vi "New TDMS Channel Group.vi"(8 "error in (no error)":errorcluster, 11 "TDMS Channel Group":T2={"Group Name"="", "Group Description"="", "Group Properties"=[], "Channels"=[], "Time Channel Options"=enum."No Time Channel", "Time Channel Name"="Time"}) -> (0 "error out":errorcluster, 3 "TdmsChannelGroup Ref":T1)   [LabVIEW 2020, in "NI_VS Data Logging API.lvlib"]
doc: "Creates a TdmsChannelGroup object based on the settings of the <b>TDMS Channel Group</b> input."
uses:
  <vilib>/NI VeriStand/Execution/DataLogging/NI_VS Data Logging API.lvlib
  <vilib>/NI VeriStand/Execution/DataLogging/TDMS Channel Group.ctl
  <vilib>/NI VeriStand/Execution/DataLogging/TDMS Property.ctl
  <vilib>/NI VeriStand/Execution/DataLogging/TDMS Channel.ctl
  <vilib>/NI VeriStand/Execution/DataLogging/Time Channel Options.ctl
  <vilib>/NI VeriStand/Execution/DataLogging/TdmsChannelGroup Ref.ctl
  NationalInstruments.VeriStand.ClientAPI
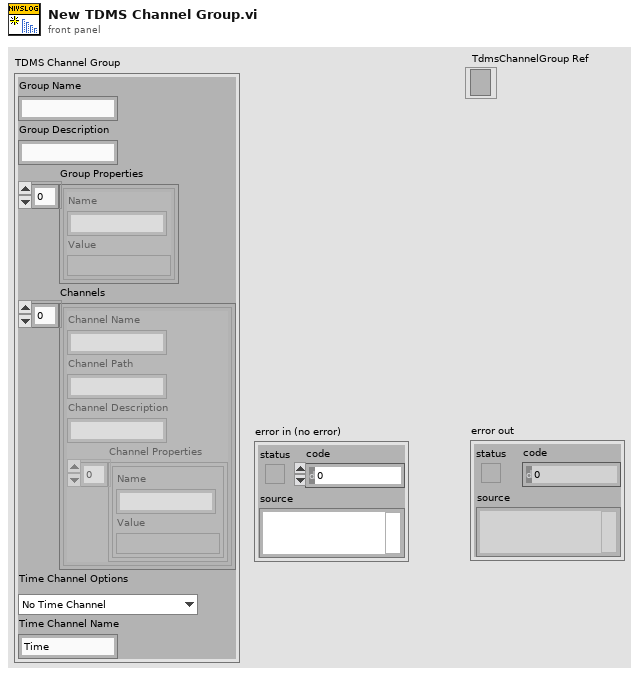
[diagram p1: front panel]
types:
  T1 = typedef "NI_VS Data Logging API.lvlib/TdmsChannelGroup Ref.ctl" = refnum<k24>
  T2 = typedef "NI_VS Data Logging API.lvlib/TDMS Channel Group.ctl" = cluster{"Group Name":string, "Group Description":string, "Group Properties":T3[], "Channels":T4[], "Time Channel Options":T5, "Time Channel Name":string}
  T3 = typedef "NI_VS Data Logging API.lvlib/TDMS Property.ctl" = cluster{"Name":string, "Value":variant}
  T4 = typedef "NI_VS Data Logging API.lvlib/TDMS Channel.ctl" = cluster{"Channel Name":string, "Channel Path":string, "Channel Description":string, "Channel Properties":T3[]}
  T5 = typedef "NI_VS Data Logging API.lvlib/Time Channel Options.ctl" = enum16{"No Time Channel", "Absolute Time", "System Time", "System Time - Microseconds", "Absolute Time as Double", "Relative To First Start Trigger", "Relative To Session Start"}
  T6 = typedef "NI_VS Data Logging API.lvlib/TdmsProperty Ref.ctl" = refnum<k24>
  T7 = typedef "NI_VS Data Logging API.lvlib/TdmsChannel Ref.ctl" = refnum<k24>
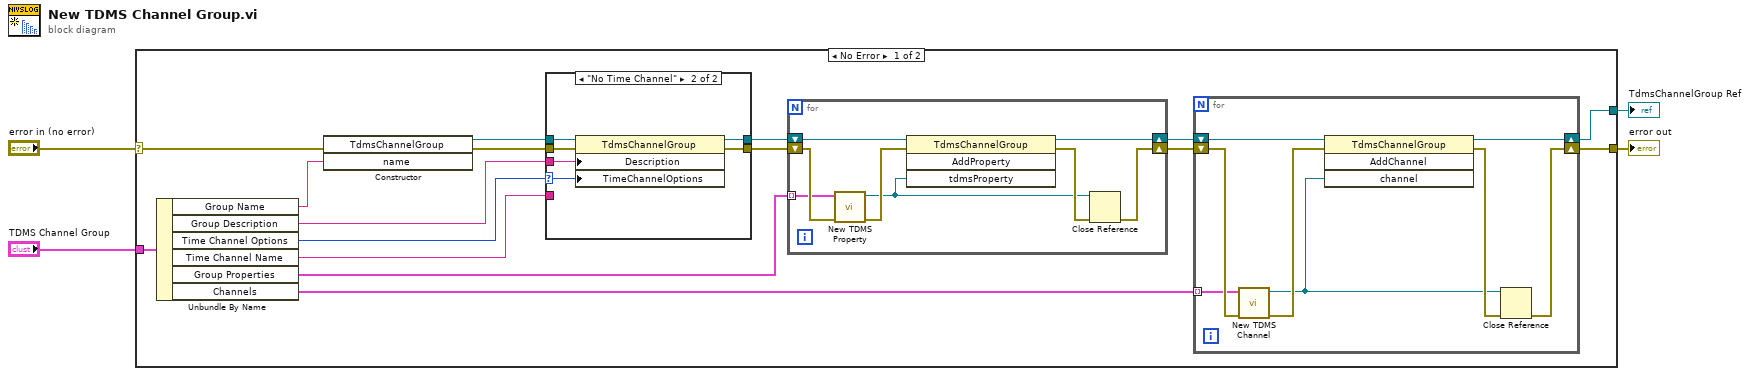
[diagram p0: block diagram]
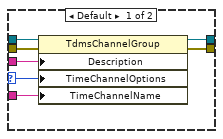
[diagram p2: hidden frame]
diagram:
  n1 = case shown="No Error" "error in (no error)" {
    selector: "error in (no error)" -> [w20 w50]
    tunnel: [w8 w50] -> w3
    tunnel: "TDMS Channel Group" -> [w19 _]
    tunnel: [w7 _] -> w1
    frame No Error {
      n2 = Unbundle By Name(w19) -> ("Group Name"=w18:string, "Group Description"=w15:string, "Time Channel Options"=w5:T5, "Time Channel Name"=w6:string, "Group Properties"=w12:T3[], "Channels"=w9:T4[])
      n3 = constructor class="TdmsChannelGroup"(error in=w20, "name"=w18) -> (reference out=w17:refnum<k24>, error out=w16:errorcluster)  [unwired: 2 in, 2 out]
      n4 = case shown="\"No Time Channel\"" w5 {
        selector: w5 -> [w21 w28]
        tunnel: w17 -> [w27 w33]
        tunnel: w16 -> [w26 w32]
        tunnel: w15 -> [w25 w31]
        tunnel: [w24 w30] -> w14
        tunnel: [w23 w29] -> w13
        tunnel: w6 -> [w22 _]
        frame Default {
          n5 = property class="TdmsChannelGroup"(reference=w27, error in=w26, "Description"=w25, "TimeChannelOptions"=w21, "TimeChannelName"=w22) -> (reference out=w24:refnum<k24>, error out=w23:errorcluster)
        }
        frame "No Time Channel" {
          n6 = property class="TdmsChannelGroup"(reference=w33, error in=w32, "Description"=w31, "TimeChannelOptions"=w28) -> (reference out=w30:refnum<k24>, error out=w29:errorcluster)
        }
      }
      n7 = for {
        tunnel: w12 -> [w45] mode=indexing
        shift-right: [w46] -> w11
        shift-left: w14 -> [w47]
        shift-right: [w42] -> w10
        shift-left: w13 -> [w48]
        n8 = call <vilib>:"New TDMS Property.vi"("error in (no error)"=w48, "TDMS Property"=w45) -> ("error out"=w49:errorcluster, "TDMSProperty Ref"=w43:T6)  [unwired: 8 in]
        n9 = invoke class="TdmsChannelGroup" method="AddProperty"(reference=w47, error in=w49, "tdmsProperty"=w43) -> (reference out=w46:refnum<k24>, error out=w44:errorcluster)  [unwired: 1 in, 2 out]
        n10 = Close Reference(reference=w43, error in (no error)=w44) -> (error out=w42:errorcluster)
      }
      n11 = for {
        shift-right: [w38] -> w7
        shift-left: w11 -> [w39]
        shift-right: [w34] -> w8
        shift-left: w10 -> [w41]
        tunnel: w9 -> [w37] mode=indexing
        n12 = call <vilib>:"New TDMS Channel.vi"("error in (no error)"=w41, "TDMS Channel"=w37) -> ("error out"=w36:errorcluster, "TdmsChannel Ref"=w35:T7)  [unwired: 8 in]
        n13 = invoke class="TdmsChannelGroup" method="AddChannel"(reference=w39, error in=w36, "channel"=w35) -> (reference out=w38:refnum<k24>, error out=w40:errorcluster)  [unwired: 1 in, 2 out]
        n14 = Close Reference(reference=w35, error in (no error)=w40) -> (error out=w34:errorcluster)
      }
    }
    frame Error {
    }
  }
  "TdmsChannelGroup Ref" <- w1
  "error out" <- w3
